vi "Trav-Positon-Info.vi"() -> ()   [LabVIEW 2017]
uses:
  TypeDefs/Position-Info-TD.ctl
panel:
  in  "Position Info":T1
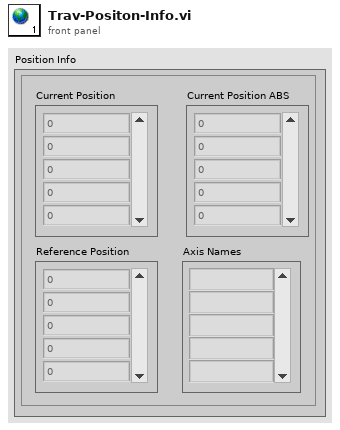
[diagram p1: front panel]
types:
  T1 = typedef "Position-Info-TD.ctl" = cluster{"Current Position ABS":dbl[], "Current Position":dbl[], "Reference Position":dbl[], "Axis Names":string[]}
diagram:
